vi "statistics.vi"() -> ()   [LabVIEW 2015]
uses:
  globalVarSD.vi
  <vilib>/Analysis/NI_AALBase.lvlib
panel:
  out "x/y":dbl
  out "Glissière":u8(slide) scale=0.0..100.0
  in  "Num":dbl
  in  "intervals":i32=10
  out "I channel RAW":cluster{i32[], "out array":dbl[]}[](graph)
  in  "wavelength":dbl
  out "II channel":T1(graph)
  out "I channel":T1(graph)
  in  "number of aq":i32=1
  in  "Measure  distribution":bool
  in  "stop":bool
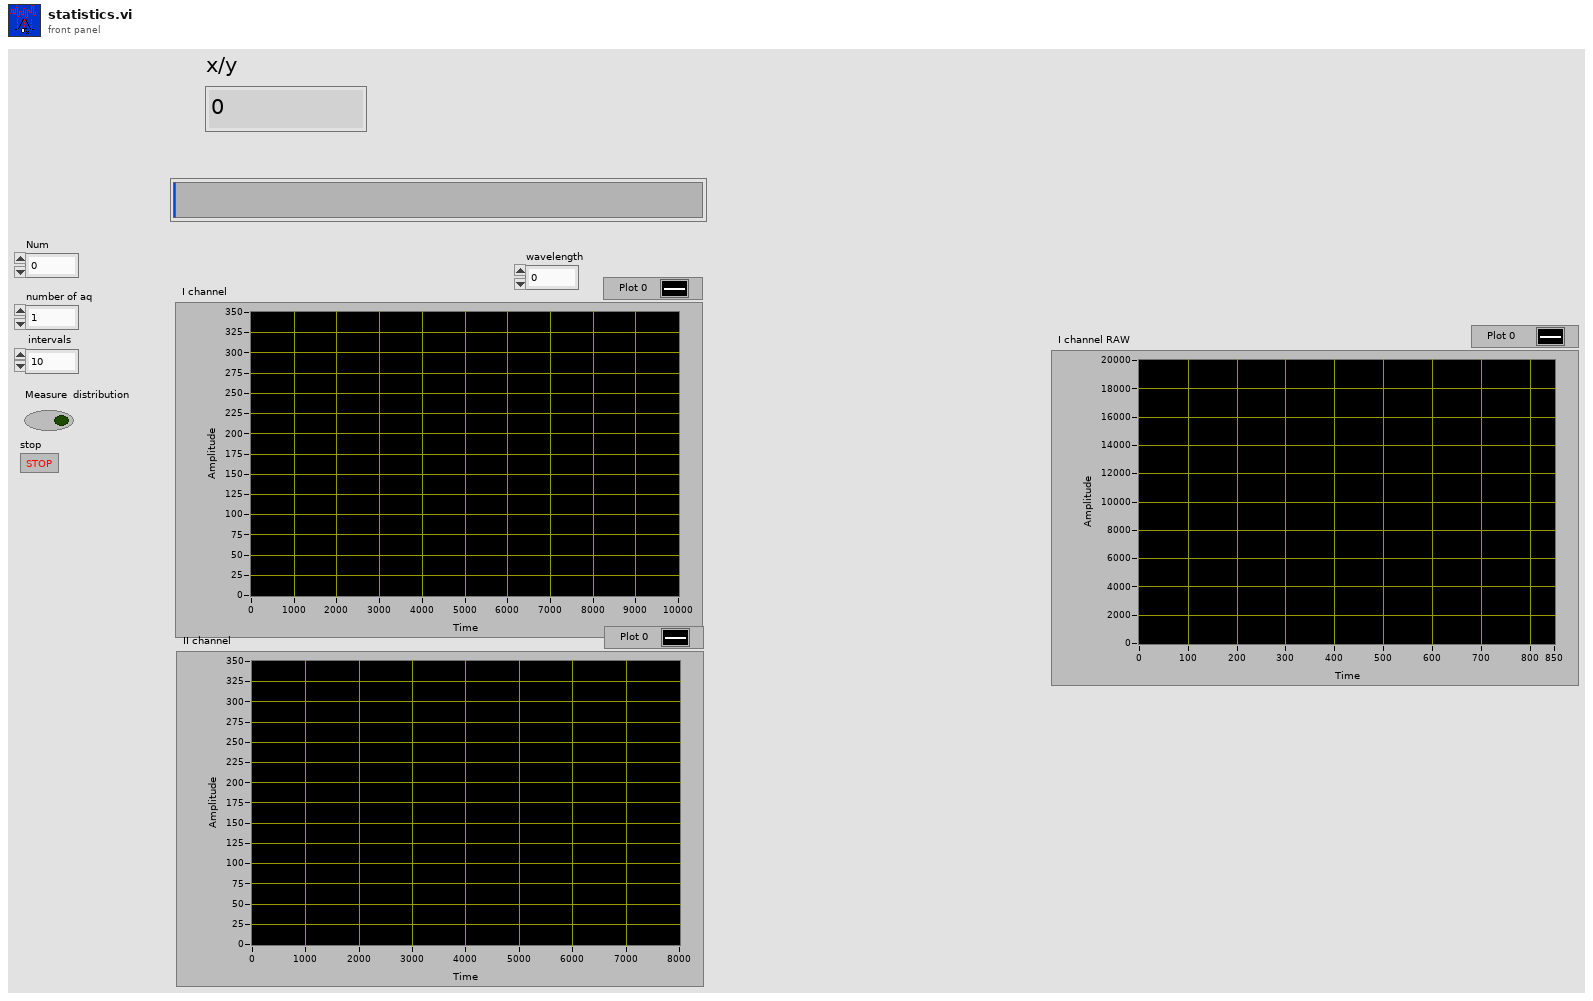
[diagram p1: front panel]
types:
  T1 = cluster{"X Values":dbl[], "Histogram: h(x)":i32[]}
  T2 = typedef "data-cluster.ctl" = cluster{"BG":i32[], "Ie":i32[], "I0":i32[]}[]
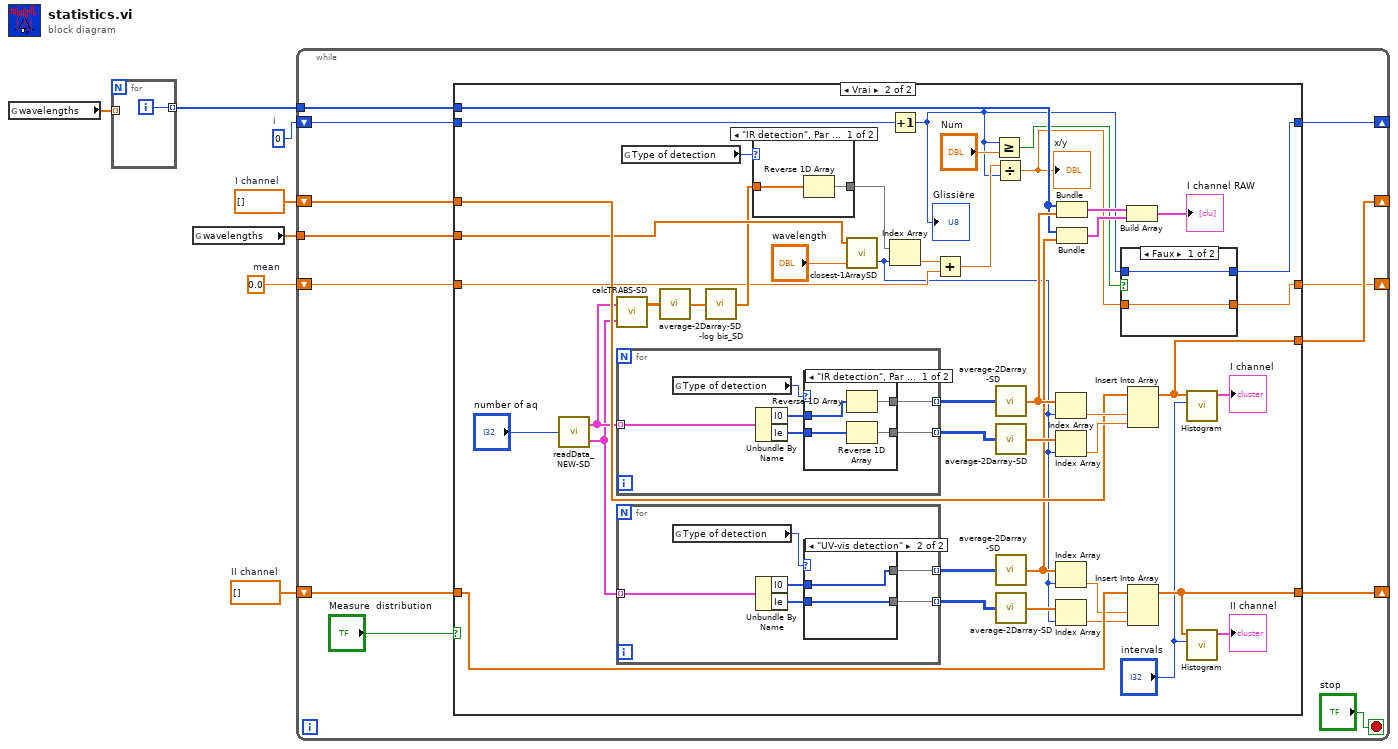
[diagram p0: block diagram]
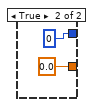
[diagram p3: hidden frame]
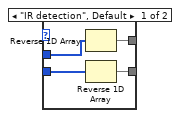
[diagram p5: hidden frame]
diagram:
  w1 = 0  # i
  w2 = 0.0  # mean
  w6 = dbl[] []  # II channel
  w7 = dbl[] []  # I channel
  n1 = global read "globalVarSD.vi" "wavelengths"() -> (w5:dbl[])
  n2 = for {
    tunnel: w5 -> [_] mode=indexing
    tunnel: [w8] -> w4 mode=indexing
    i -> [w8]
  }
  n3 = global read "globalVarSD.vi" "wavelengths"() -> (w3:dbl[])
  n4 = while {
    shift-right: [w18] -> _
    shift-left: w7 -> [w17]
    shift-right: [w16] -> _
    shift-left: w6 -> [w15]
    tunnel: w4 -> [w14]
    tunnel: w3 -> [w13]
    shift-right: [w11] -> _
    shift-left: w2 -> [w12]
    shift-right: [w9] -> _
    shift-left: w1 -> [w10]
    stop <- "stop" stop-if-true
    n5 = case shown="Vrai" "Measure  distribution" {
      tunnel: [w24 w49] -> w18
      tunnel: w17 -> [w24 w55]
      tunnel: [w23 w50] -> w16
      tunnel: w15 -> [w23 w54]
      tunnel: w14 -> [_ w45]
      tunnel: w13 -> [_ w44]
      tunnel: w12 -> [w22 w34]
      tunnel: w10 -> [w21 w33]
      tunnel: [w21 w29] -> w9
      tunnel: [w22 w27] -> w11
      frame False {
      }
      frame True {
        n6 = call "readData_NEW-SD.vi"("number of aq"="number of aq") -> ("I channel seq"=w39:T2, "II channel seq"=w38:T2)
        n7 = call "calcTRABS-SD.vi"("II channel seq"=w38, "I channel seq"=w39) -> ("TRanS multiple measurements"=w40:dbl[][])  [unwired: 1 out]
        n8 = for {
          tunnel: w39 -> [w93] mode=indexing
          tunnel: [w90] -> w65 mode=indexing
          tunnel: [w89] -> w64 mode=indexing
          n9 = global read "globalVarSD.vi" "Type of detection"() -> (w88:enum32{"IR detection", "UV-vis detection"})
          n10 = Unbundle By Name(w93) -> ("I0"=w91:i32[], "Ie"=w92:i32[])
          n11 = case shown="\"IR detection\", Par défaut" w88 {
            tunnel: w91 -> [w97 w99]
            tunnel: [w96 w99] -> w90
            tunnel: [w95 w98] -> w89
            tunnel: w92 -> [w94 w98]
            frame "IR detection", Default {
              n12 = Reverse 1D Array(array=w97) -> (reversed array=w96:i32[])
              n13 = Reverse 1D Array(array=w94) -> (reversed array=w95:i32[])
            }
            frame "UV-vis detection" {
            }
          }
        }
        n14 = for {
          tunnel: w38 -> [w81] mode=indexing
          tunnel: [w78] -> w61 mode=indexing
          tunnel: [w76] -> w62 mode=indexing
          n15 = global read "globalVarSD.vi" "Type of detection"() -> (w80:enum32{"IR detection", "UV-vis detection"})
          n16 = Unbundle By Name(w81) -> ("I0"=w79:i32[], "Ie"=w77:i32[])
          n17 = case shown="\"UV-vis detection\"" w80 {
            tunnel: w79 -> [w85 w87]
            tunnel: [w84 w87] -> w78
            tunnel: w77 -> [w83 w86]
            tunnel: [w82 w86] -> w76
            frame "IR detection", Default {
              n18 = Reverse 1D Array(array=w85) -> (reversed array=w84:i32[])
              n19 = Reverse 1D Array(array=w83) -> (reversed array=w82:i32[])
            }
            frame "UV-vis detection" {
            }
          }
        }
        n20 = global read "globalVarSD.vi" "Type of detection"() -> (w43:enum32{"IR detection", "UV-vis detection"})
        n21 = call "average-2Darray-SD.vi"("2D array"=w40) -> ("out array"=w41:dbl[])
        n22 = call "-log bis_SD.vi"("Transmission"=w41) -> ("-log(x)=log(1/x)"=w42:dbl[])
        n23 = case shown="\"IR detection\", Par défaut" w43 {
          tunnel: w42 -> [w74 w75]
          tunnel: [w73 w75] -> w37
          frame "IR detection", Default {
            n24 = Reverse 1D Array(array=w74) -> (reversed array=w73:dbl[])
          }
          frame "UV-vis detection" {
          }
        }
        n25 = call "closest-1ArraySD.vi"("desired element"="wavelength", "1D Array"=w44) -> ("closest index"=w25:i32)  [unwired: 1 in, 1 out]
        n26 = Increment(x=w33) -> (x+1=w26:i32)
        "Glissière" <- w26
        n27 = Index Array(array=w37, index=w25) -> (element=w35:dbl)
        n28 = Add(x=w35, y=w34) -> (x+y=w32:dbl)
        n29 = Greater Or Equal?(x=w26, y="Num") -> (x >= y?=w30:bool)
        n30 = Divide(x=w32, y=w26) -> (x/y=w28:dbl)
        "x/y" <- w28
        n31 = call "average-2Darray-SD.vi"("2D array"=w65) -> ("out array"=w47:dbl[])
        n32 = call "average-2Darray-SD.vi"("2D array"=w64) -> ("out array"=w63:dbl[])
        n33 = call "average-2Darray-SD.vi"("2D array"=w61) -> ("out array"=w46:dbl[])
        n34 = call "average-2Darray-SD.vi"("2D array"=w62) -> ("out array"=w52:dbl[])
        n35 = Index Array(array=w47, index=w25) -> (element=w57:dbl)
        n36 = Index Array(array=w63, index=w25) -> (element=w56:dbl)
        n37 = Index Array(array=w46, index=w25) -> (element=w53:dbl)
        n38 = Index Array(array=w52, index=w25) -> (element=w51:dbl)
        n39 = Bundle(w45, "out array"=w47) -> (w60:cluster{i32[], "out array":dbl[]})  [unwired: 1 in]
        n40 = Bundle(w45, "out array"=w46) -> (w59:cluster{i32[], "out array":dbl[]})  [unwired: 1 in]
        n41 = case shown="Faux" w30 {
          tunnel: w26 -> [w70 _]
          tunnel: [w70 0] -> w29
          tunnel: w28 -> [w69 _]
          tunnel: [w69 0.0] -> w27
          frame False {
          }
          frame True {
          }
        }
        n42 = Build Array(w60, w59) -> (→"I channel RAW":cluster{i32[], "out array":dbl[]}[])
        n43 = Insert Into Array(array=w55, new element #1=w57, new element #2=w56) -> (w49:dbl[])  [unwired: 1 in]
        n44 = Insert Into Array(array=w54, new element #1=w53, new element #2=w51) -> (w50:dbl[])  [unwired: 1 in]
        n45 = call <vilib>:"Histogram.vi"("intervals"="intervals", "X"=w49) -> ("Histogram Graph"=→"I channel":T1)  [unwired: 6 in, 3 out]
        n46 = call <vilib>:"Histogram.vi"("intervals"="intervals", "X"=w50) -> ("Histogram Graph"=→"II channel":T1)  [unwired: 6 in, 3 out]
      }
    }
  }
